vi "Check for changed Items and update tree.vi"(8 "error in":errorcluster, 11 "Configuration":T1={"Data Tree Ref"=refnum, "FP Ref"=refnum, "Column Data Type"=[], "Search Clones Up To"=0, "SortOptions"={"Col.pri"=0, "RevDir.pri"=FALSE, "Col.sec"=0, "RevDir.sec"=FALSE}, "Group/Flat (0:group)"=FALSE, "CollapsedNodes"=[], "Show/Hide Cols"=[], "Filtered Paths"=[], "View"=enum."Group By Library", "File Extension Filters"=[], "Filter Global VIs"=FALSE, "Shared"=refnum, "Active Filters"=refnum, "Refresh Rate (ms)"=2000}) -> (0 "error out":errorcluster)   [LabVIEW 2013, in "LVTM.lvlib"]
uses:
  LVTM.lvlib
  Controls_LVTM/LVTM_Config_Info.ctl
  Controls_LVTM/View.ctl
  Controls_LVTM/SharedDataDVR.ctl
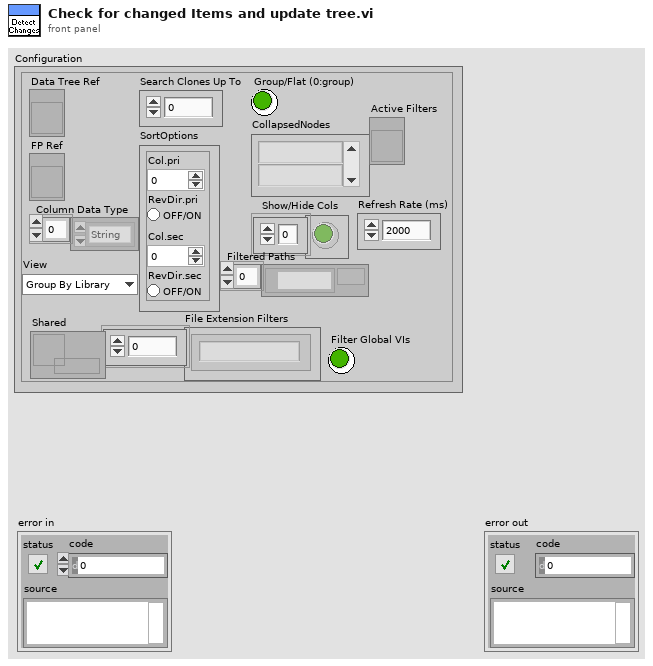
[diagram p1: front panel]
types:
  T1 = typedef "LVTM.lvlib/LVTM_Config_Info.ctl" = cluster{"Data Tree Ref":refnum<vi>, "FP Ref":refnum<vi>, "Column Data Type":enum16{"String", "Numeric"}[], "Search Clones Up To":i32, "SortOptions":cluster{"Col.pri":i32, "RevDir.pri":bool, "Col.sec":i32, "RevDir.sec":bool}, "Group/Flat (0:group)":bool, "CollapsedNodes":string[], "Show/Hide Cols":bool[], "Filtered Paths":path[], "View":T2, "File Extension Filters":string[], "Filter Global VIs":bool, "Shared":refnum<data-value>, "Active Filters":refnum<vi>, "Refresh Rate (ms)":i32}
  T2 = typedef "LVTM.lvlib/View.ctl" = enum16{"Group By Library", "Group By Folder", "Flat List"}
  T3 = typedef "LVTM.lvlib/SharedDataDVR.ctl" = cluster{"App":refnum<vi>, "VIs":string[]}
  T4 = cluster{"Item Tag":string, "Column":i32[], "Value":string[]}[]
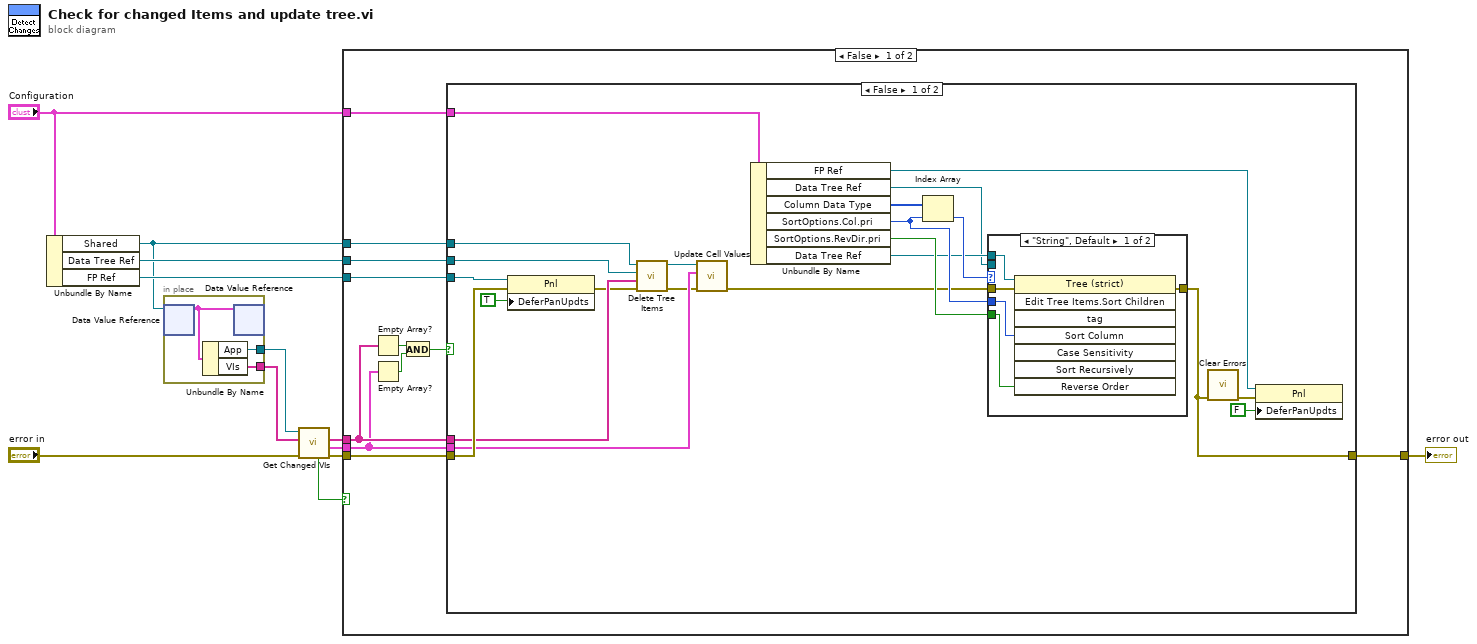
[diagram p0: block diagram]
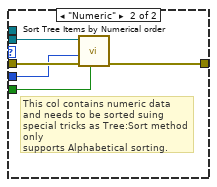
[diagram p2: hidden frame]
diagram:
  n1 = Unbundle By Name("Configuration") -> ("Shared"=w4:refnum<data-value>, "Data Tree Ref"=w11:refnum<vi>, "FP Ref"=w10:refnum<vi>)
  n2 = in-place {
    in-place-border: [w14] -> w8
    in-place-border: [w13] -> w7
    n3 = in-place-dvr #1(w4) -> (w15:T3)  [unwired: 1 out]
    n4 = Unbundle By Name(w15) -> ("App"=w14:refnum<vi>, "VIs"=w13:string[])
    n5 = in-place-dvr #1(w15) -> ()  [unwired: 2 out]
  }
  n6 = call "Get Changed VIs.vi"("error in"="error in", "VIs"=w7, "Application in"=w8) -> ("error out"=w2:errorcluster, "Changed Items"=w5:T4, "Items no longer in memory"=w6:string[], "Canceled"=w1:bool)  [unwired: 5 in]
  n7 = case shown="False" w1 {
    tunnel: "Configuration" -> [w26 _]
    tunnel: w11 -> [w25 _]
    tunnel: w10 -> [w24 _]
    tunnel: [w23 w60] -> w9
    tunnel: w6 -> [w20 _]
    tunnel: w5 -> [w19 _]
    tunnel: w4 -> [w22 _]
    tunnel: w2 -> [w21 w60]
    frame False {
      n8 = Empty Array?(array=w20) -> (empty?=w18:bool)
      n9 = Empty Array?(array=w19) -> (empty?=w17:bool)
      n10 = And(x=w18, y=w17) -> (x .and. y?=w16:bool)
      n11 = case shown="False" w16 {
        tunnel: w26 -> [w47 _]
        tunnel: w25 -> [w46 _]
        tunnel: w24 -> [w45 _]
        tunnel: [w32 w59] -> w23
        tunnel: w22 -> [w37 _]
        tunnel: w21 -> [w35 w59]
        tunnel: w20 -> [w34 _]
        tunnel: w19 -> [w33 _]
        frame False {
          n12 = property class="Pnl"(reference=w45, error in=w35, "DeferPanUpdts"=TRUE ("Defer Panel Updates")) -> (error out=w30:errorcluster)  [unwired: 1 out]
          n13 = call "Delete Tree Items.vi"("error in (no error)"=w30, "Items no longer in memory"=w34, "Data Tree Ref"=w46, "Data Value Reference in"=w37) -> ("error out"=w29:errorcluster, "TreeControl out"=w28:refnum<vi>)  [unwired: 6 in]
          n14 = call "Update Cell Values.vi"("error in (no error)"=w29, "Changed Items"=w33, "TreeControl in"=w28) -> ("error out"=w27:errorcluster)  [unwired: 8 in]
          n15 = Unbundle By Name(w47) -> ("FP Ref"=w48:refnum<vi>, "Data Tree Ref"=w36:refnum<vi>, "Column Data Type"=w41:enum16{"String", "Numeric"}[], "SortOptions.Col.pri"=w42:i32, "SortOptions.RevDir.pri"=w43:bool, "Data Tree Ref"=w38:refnum<vi>)
          n16 = Index Array(array=w41, index=w42) -> (element=w44:enum16{"String", "Numeric"})
          n17 = case shown="\"String\", Default" w44 {
            tunnel: [w53 w57] -> w32
            tunnel: w43 -> [w52 w56]
            tunnel: w27 -> [w51 w58]
            tunnel: w42 -> [w50 w54]
            tunnel: w36 -> [_ w55]
            tunnel: w38 -> [w49 _]
            frame "String", Default {
              n18 = invoke on="Invoke Node" class="Tree (strict)" method="Edit Tree Items.Sort Children"(reference=w49, error in=w51, "Sort Column"=w50, "Reverse Order"=w52) -> (error out=w53:errorcluster)  [unwired: 4 in, 7 out]
            }
            frame "Numeric" {
              # "This col contains numeric data and needs to be sorted suing special tricks as Tree:Sort method only\nsupports Alphabetical sorting."
              n19 = call "Sort Tree Items by Numerical order.vi"("Reverse Order?"=w56, "error in"=w58, "Sort Column"=w54, "Data Tree"=w55) -> ("error out"=w57:errorcluster)  [unwired: 7 in]
            }
          }
          n20 = call <vilib>:"Clear Errors.vi"("error in (no error)"=w32) -> ("error out"=w31:errorcluster)  [unwired: 6 in]
          n21 = property class="Pnl"(reference=w48, error in=w31, "DeferPanUpdts"=FALSE ("Defer Panel Updates")) -> ()  [unwired: 2 out]
        }
        frame True {
        }
      }
    }
    frame True {
    }
  }
  "error out" <- w9
